vi "Get Label Properties.vi"(8 "error in":errorcluster, 11 "label ref in":T3 format="%.0x") -> (0 "error out":errorcluster, 2 "label properties":T1, 3 "label ref out":T3 format="%.0x", 4 "found?":bool)   [LabVIEW 2020, in "ARINC 429 Scripting.lvlib"]
uses:
  ARINC 429 Scripting.lvlib
  <vilib>/NI VeriStand/Custom Device API/Custom Device Item Ref.ctl
  Shared/Label Properties.ctl
  Shared/Label.ctl
  Constants.vi
  <vilib>/NI VeriStand/Custom Device API/Get Item Property (U32).vi
  <vilib>/NI VeriStand/Custom Device API/Get Item Property (U16).vi
  <vilib>/NI VeriStand/Custom Device API/Get Item Property (Boolean).vi
  <vilib>/NI VeriStand/Custom Device API/Custom Device API.lvlib
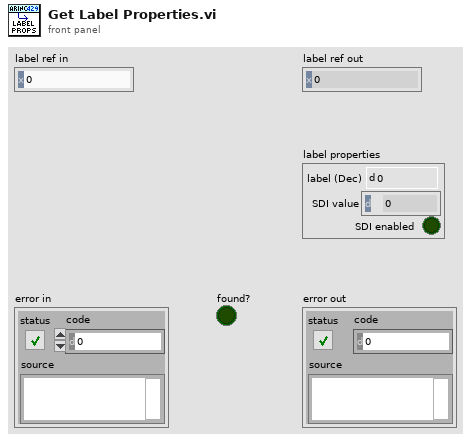
[diagram p1: front panel]
types:
  T1 = typedef "Label Properties.ctl" = cluster{"label (Dec)":T2, "SDI value":u8, "SDI enabled":bool}
  T2 = typedef "Label.ctl" = u8
  T3 = typedef "Custom Device API.lvlib/Custom Device Item Ref.ctl" = u64
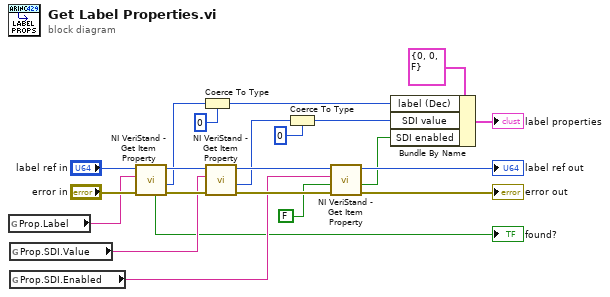
[diagram p0: block diagram]
diagram:
  n1 = global read "Constants.vi" "Prop.Label"() -> (w12:string)
  n2 = global read "Constants.vi" "Prop.SDI.Value"() -> (w11:string)
  n3 = global read "Constants.vi" "Prop.SDI.Enabled"() -> (w14:string)
  n4 = call-poly <vilib>:"NI VeriStand - Get Item Property.vi"("error in (no error)"="error in", "Property Name"=w12, "Item Ref in"="label ref in") -> ("error out"=w17:errorcluster, "Value"=w2:u32, "Item Ref out"=w18:T3, "Found?"=→"found?":bool)  [unwired: 5 in]
  n5 = Coerce To Type(0:w2, 1:T2 0 ("label")) -> (2:w1:T2)
  n6 = call-poly <vilib>:"NI VeriStand - Get Item Property.vi"("error in (no error)"=w17, "Property Name"=w11, "Item Ref in"=w18) -> ("error out"=w15:errorcluster, "Value"=w9:u16, "Item Ref out"=w16:T3)  [unwired: 5 in, 1 out]
  n7 = Coerce To Type(0:w9, 1:u8 0 ("SDI value")) -> (2:w8:u8)
  n8 = call-poly <vilib>:"NI VeriStand - Get Item Property.vi"("error in (no error)"=w15, "Default Value"=FALSE, "Property Name"=w14, "Item Ref in"=w16) -> ("error out"=→"error out":errorcluster, "Value"=w7:bool, "Item Ref out"=→"label ref out":T3)  [unwired: 4 in, 1 out]
  n9 = Bundle By Name(cluster=T1 {"label (Dec)"=0, "SDI value"=0, "SDI enabled"=FALSE} ("label properties"), "label (Dec)"=w1, "SDI value"=w8, "SDI enabled"=w7) -> (→"label properties":T1)
